vi "writeAIchan_string_tt.vi"() -> (0 "AI?":bool, 1 "AIChannel string":string)   [LabVIEW 2013]
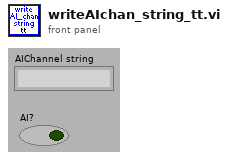
[diagram p1: front panel]
types:
  T1 = cluster{"StageS":i32, "StageL":i32, "data dir":path, "image OD":u16, "contour OD":u16, "point OD":u16, "AOlines":tag[], "AIlines":tag[], "CI lines":tag[], "DO lines":tag[], "AO names":string[], "CI names":string[], "AI names":string[], "DO names":string[], "CIextensions":string[], "AIextensions":string[], "Voltage to Ygalvo":i32, "Voltage to Xgalvo":i32, "Voltage to patch":i32, "640 shutter":i32, "2P shutter":i32, "LT timestamp":i32, "Vp":i32, "Ip":i32}
  T2 = typedef "LVRectTypeDef.ctl" = cluster{"Left":i16, "Top":i16, "Right":i16, "Bottom":i16}
  T3 = cluster{"Xpixels":i32, "Vxminref":dbl, "Vxmaxref":dbl, "P":dbl, "Ypixels":i32, "Vyminref":dbl, "Vymaxref":dbl, "srate":sgl, "sAOxy":i32, "timeout":dbl, "type":string, "date":string, "time":string, "Colormap":u16, "Drawing Mode":u16, "Scanning Mode":u16, "square pixels":bool, "square matrix":bool, "Xpixels Img":i32, "Vx-min Img":dbl, "VX-max Img":dbl, "Ypixels Img":i32, "Vy-min Img":dbl, "Vy-max Img ":dbl, "Angle Img":dbl, "autoshutter":bool, "finite":bool, "cont":bool, "wavdet":bool, "measpoints":i32, "avpp":i32, "bufferAO":i32, "bufferAI":i32, "starttick":u32, "waveform":path, "Vx-ref":dbl, "Vy-ref":dbl, "refreshrate":dbl, "refreshbuffer":i32, "tt_cycles":i32, "motorref":refnum<k7>, "mirrorswitch":refnum<k7>, "sample mode":i32, "maxbufferAI":i32, "sampletreshold":dbl, "srateAODO":sgl, "bin":sgl, "Pel":sgl, "Angle draw":dbl, "srate Img":sgl, "ROIimg_plotbounds":T2, "auto OD":bool, "ODfilt":u16, "reset AO_DO":bool, "aAI":i32[], "aCI":i32[], "aAO":i32[], "aDO":i32[]}
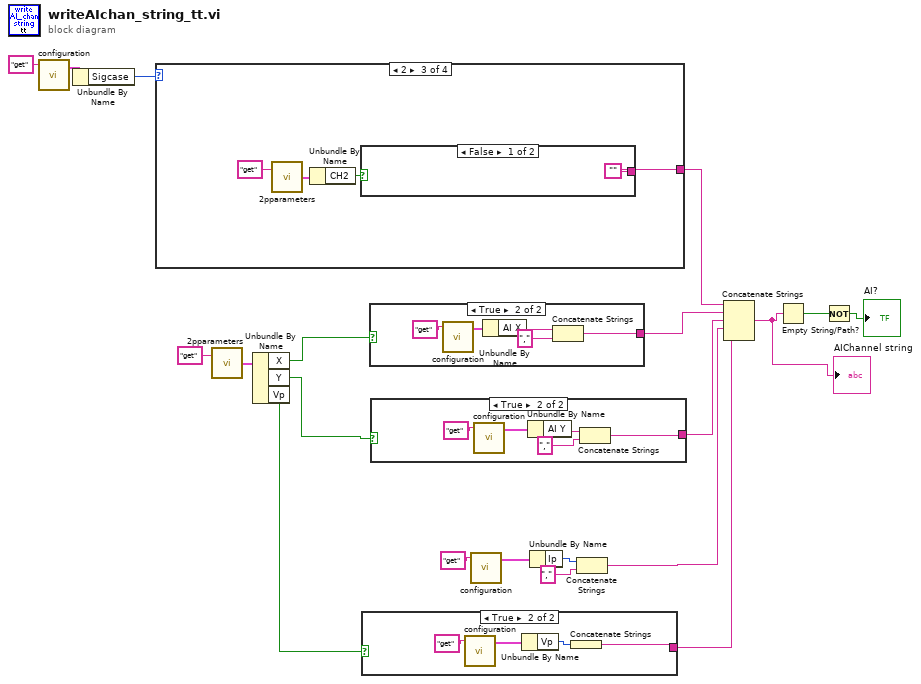
[diagram p0: block diagram]
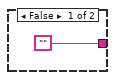
[diagram p2: hidden frame]
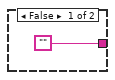
[diagram p3: hidden frame]
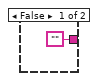
[diagram p4: hidden frame]
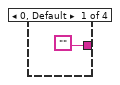
[diagram p5: hidden frame]
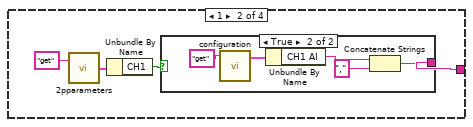
[diagram p6: hidden frame]
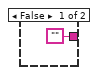
[diagram p7: hidden frame]
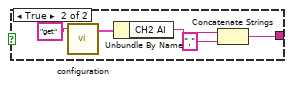
[diagram p8: hidden frame]
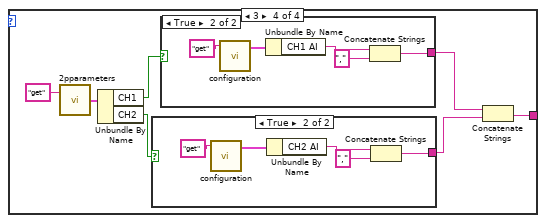
[diagram p9: hidden frame]
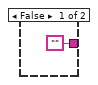
[diagram p10: hidden frame]
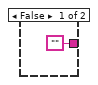
[diagram p11: hidden frame]
diagram:
  n1 = call "configuration.vi"("command"="get") -> ("config out"=w11:T1)  [unwired: 2 in, 1 out]
  n2 = Unbundle By Name(w11) -> ("Sigcase"=w12:i16)
  n3 = case shown="2" w12 {
    tunnel: ["" w22 w35 w46] -> w19
    frame 0, Default {
    }
    frame 1 {
      n4 = call "2pparameters.vi"("command"="get") -> ("params out"=w24:T3)  [unwired: 1 in]
      n5 = Unbundle By Name(w24) -> ("CH1"=w23:bool)
      n6 = case shown="True" w23 {
        tunnel: ["" w27] -> w22
        frame False {
        }
        frame True {
          n7 = call "configuration.vi"("command"="get") -> ("config out"=w30:T1)  [unwired: 2 in, 1 out]
          n8 = Unbundle By Name(w30) -> ("CH1 AI"=w31:tag)
          n9 = Concatenate Strings(w31, ",") -> (w27:string)
        }
      }
    }
    frame 2 {
      n10 = call "2pparameters.vi"("command"="get") -> ("params out"=w33:T3)  [unwired: 1 in]
      n11 = Unbundle By Name(w33) -> ("CH2"=w32:bool)
      n12 = case shown="False" w32 {
        tunnel: ["" w37] -> w35
        frame False {
        }
        frame True {
          n13 = call "configuration.vi"("command"="get") -> ("config out"=w40:T1)  [unwired: 2 in, 1 out]
          n14 = Unbundle By Name(w40) -> ("CH2 AI"=w41:tag)
          n15 = Concatenate Strings(w41, ",") -> (w37:string)
        }
      }
    }
    frame 3 {
      n16 = call "2pparameters.vi"("command"="get") -> ("params out"=w44:T3)  [unwired: 1 in]
      n17 = Unbundle By Name(w44) -> ("CH1"=w43:bool, "CH2"=w42:bool)
      n18 = case shown="True" w42 {
        tunnel: ["" w50] -> w47
        frame False {
        }
        frame True {
          n19 = call "configuration.vi"("command"="get") -> ("config out"=w53:T1)  [unwired: 2 in, 1 out]
          n20 = Unbundle By Name(w53) -> ("CH2 AI"=w54:tag)
          n21 = Concatenate Strings(w54, ",") -> (w50:string)
        }
      }
      n22 = case shown="True" w43 {
        tunnel: ["" w56] -> w48
        frame False {
        }
        frame True {
          n23 = call "configuration.vi"("command"="get") -> ("config out"=w59:T1)  [unwired: 2 in, 1 out]
          n24 = Unbundle By Name(w59) -> ("CH1 AI"=w60:tag)
          n25 = Concatenate Strings(w60, ",") -> (w56:string)
        }
      }
      n26 = Concatenate Strings(w48, w47) -> (w46:string)
    }
  }
  n27 = call "2pparameters.vi"("command"="get") -> ("params out"=w15:T3)  [unwired: 1 in]
  n28 = Unbundle By Name(w15) -> ("X"=w14:bool, "Y"=w13:bool, "Vp"=w9:bool)
  n29 = case shown="True" w9 {
    tunnel: ["" w62] -> w7
    frame False {
    }
    frame True {
      n30 = call "configuration.vi"("command"="get") -> ("config out"=w64:T1)  [unwired: 2 in, 1 out]
      n31 = Unbundle By Name(w64) -> ("Vp"=w65:i32)
      n32 = Concatenate Strings(w65) -> (w62:string)
    }
  }
  n33 = case shown="True" w14 {
    tunnel: ["" w67] -> w17
    frame False {
    }
    frame True {
      n34 = call "configuration.vi"("command"="get") -> ("config out"=w70:T1)  [unwired: 2 in, 1 out]
      n35 = Unbundle By Name(w70) -> ("AI X"=w71:tag)
      n36 = Concatenate Strings(w71, ",") -> (w67:string)
    }
  }
  n37 = case shown="True" w13 {
    tunnel: ["" w74] -> w18
    frame False {
    }
    frame True {
      n38 = call "configuration.vi"("command"="get") -> ("config out"=w76:T1)  [unwired: 2 in, 1 out]
      n39 = Unbundle By Name(w76) -> ("AI Y"=w77:tag)
      n40 = Concatenate Strings(w77, ",") -> (w74:string)
    }
  }
  n41 = call "configuration.vi"("command"="get") -> ("config out"=w3:T1)  [unwired: 2 in, 1 out]
  n42 = Unbundle By Name(w3) -> ("Ip"=w4:i32)
  n43 = Concatenate Strings(w4, ",") -> (w8:string)
  n44 = Concatenate Strings(w19, w17, w18, w8, w7) -> (w6:string)
  "AIChannel string" <- w6
  n45 = Empty String/Path?(string/path=w6) -> (empty?=w20:bool)
  n46 = Not(x=w20) -> (.not. x?=→"AI?":bool)
